vi "Init Hardware.vi"(8 "error in (no error)":errorcluster, 11 "RP I-V Driver in":refnum<class "RP I-V Driver.lvclass">) -> (0 "error out":errorcluster, 3 "RP I-V Driver out":refnum<class "RP I-V Driver.lvclass">)   [LabVIEW 2016, in "RP I-V Driver.lvclass"]
uses:
  RP I-V Driver.lvclass
  C:/github/NHMFL_Core/Libraries/Red Pitaya/Red Pitaya Digitizer/Red Pitaya Digitizer.lvclass
  C:/github/NHMFL_Core/Libraries/Instruments/Pulse Driver/Pulse Driver.lvclass
  RP Command.ctl
  Red Pitaya Digitizer/Red Pitaya Digitizer.lvclass/Red Pitaya Digitizer.ctl
  Instruments/Pulse Driver/Pulse Driver.lvclass/Pulse Driver.ctl
  RP I-V Driver.lvclass/RP I-V Driver.ctl
  Red Pitaya Digitizer/Read RP Instrument.vi
  Instruments/Pulse Driver/Read Scaling coefficients.vi
  Red Pitaya Digitizer/Write RP Instrument.vi
  Write Output waveform.vi
  Instruments/Pulse Driver/Write Scaling coefficients.vi
  Red Pitaya Digitizer/Red Pitaya Digitizer.lvclass
  RP Instrument/RP Instrument.lvclass
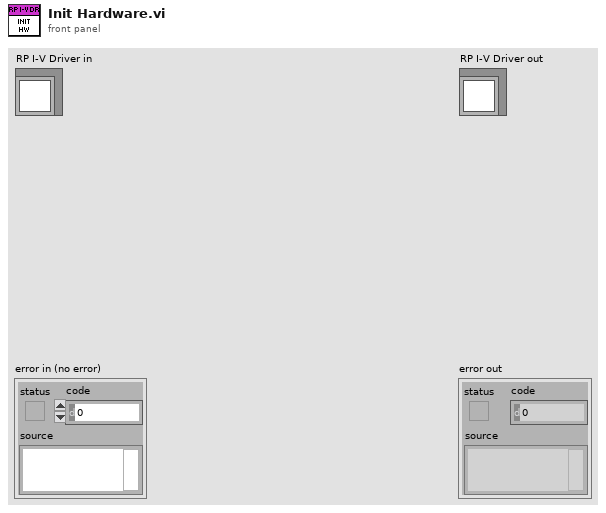
[diagram p1: front panel]
types:
  T1 = typedef "RP Command.ctl" = enum16{"Reset", "Read IDN", "Stop server", "Get status", "Get temperature", "Connect client", "Arm", "Software trigger", "Get whole buffer", "Get chunk", "System call", "Get config", "Set config", "Recieve data", "Recieve Calibartion", "Transmit data"}
  T2 = typedef "RP I-V Configuration.ctl" = cluster{"I-V parameters":T3, "Ranges":dbl[], "Pre-trigger duration":dbl, "Post-trigger duration":dbl, "Output delay":dbl}
  T3 = typedef "I-V parameters.ctl" = cluster{"Start magnitude":dbl, "Magnitude increment":dbl, "End magnitude":dbl, "Baseline length":i32, "Ramp length":i32, "Top  length":i32, "Threshold ":dbl, "Processing delay":u16, "Valhalla range":dbl, "Interpolation":i32, "Stop after":u16}
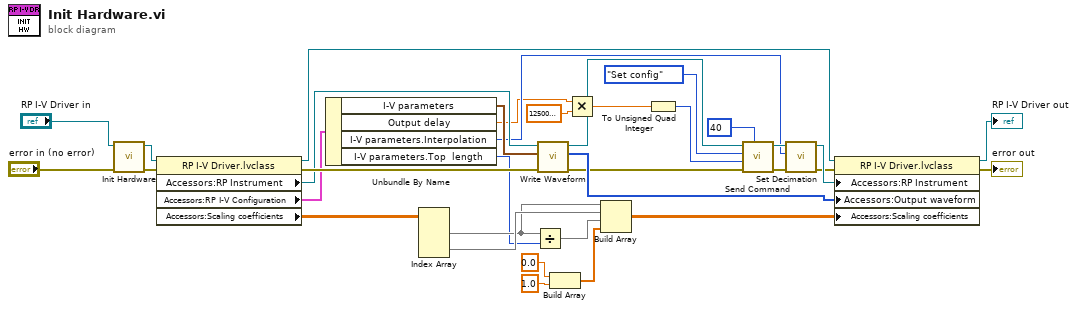
[diagram p0: block diagram]
diagram:
  n1 = call-parent "Init Hardware.vi"("error in (no error)"="error in (no error)", "Red Pitaya Digitizer in"="RP I-V Driver in") -> ("error out"=w19:errorcluster, "Red Pitaya Digitizer out"=w18:refnum<class "RP I-V Driver.lvclass">)  [unwired: 8 in]
  n2 = property class="RP I-V Driver.lvclass"(reference=w18, error in=w19) -> (reference out=w34:refnum<class "RP I-V Driver.lvclass">, error out=w33:errorcluster, "Accessors:RP Instrument"=w32:refnum<class "RP Instrument.lvclass">, "Accessors:RP I-V Configuration"=w26:T2, "Accessors:Scaling coefficients"=w10:dbl[][])
  n3 = Unbundle By Name(w26) -> ("I-V parameters"=w25:T3, "Output delay"=w1:dbl, "I-V parameters.Interpolation"=w11:i32, "I-V parameters.Top  length"=w7:i32)
  n4 = Index Array(array=w10) -> (element #1=w8:dbl[], element #2=w9:dbl[])  [unwired: 4 in]
  n5 = Divide(x=w8, y=w7) -> (x/y=w6:dbl[])
  n6 = call-dynamic "Write Waveform.vi"("error in (no error)"=w33, "I-V parameters"=w25, "RP Instrument in"=w32) -> ("error out"=w29:errorcluster, "Output Waveform"=w31:i16[], "RP Instrument out"=w30:refnum<class "RP Instrument.lvclass">)  [unwired: 6 in]
  n7 = Build Array(0.0 ("element"), 1.0 ("element")) -> (w3:dbl[])
  n8 = Multiply(x=w1, y=125000000.0) -> (x*y=w23:dbl)
  n9 = Build Array(w8, w9, w6, w3) -> (w2:dbl[][])
  n10 = To Unsigned Quad Integer(1:w23) -> (0:w22:u64)
  n11 = call-dynamic "Send Command.vi"("Config offset"=u64 40, "error in (no error)"=w29, "Command payload"=w22, "Command number"=RP_Command."Set config", "RP Instrument in"=w30) -> ("error out"=w13:errorcluster, "RP Instrument out"=w15:refnum<class "RP Instrument.lvclass">)  [unwired: 5 in]
  n12 = call-dynamic "Set Decimation.vi"("error in (no error)"=w13, "Decimation"=w11, "RP Instrument in"=w15) -> ("error out"=w12:errorcluster, "RP Instrument out"=w14:refnum<class "RP Instrument.lvclass">)  [unwired: 7 in]
  n13 = property class="RP I-V Driver.lvclass"(reference=w34, error in=w12, "Accessors:RP Instrument"=w14, "Accessors:Output waveform"=w31, "Accessors:Scaling coefficients"=w2) -> (reference out=→"RP I-V Driver out":refnum<class "RP I-V Driver.lvclass">, error out=→"error out":errorcluster)
